vi "Test PrintWithReturn 2.vi"() -> ()   [LabVIEW 2014, in "Arduino SoftwareSerial Wrapper.lvlib"]
uses:
  Arduino SoftwareSerial Wrapper.lvlib
panel:
  out "Bytes written":u8
  out "Error Out":errorcluster
  in  "Error In":errorcluster
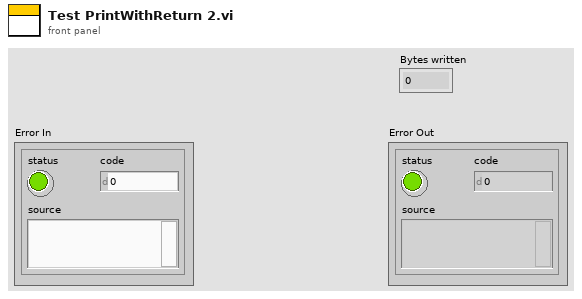
[diagram p1: front panel]
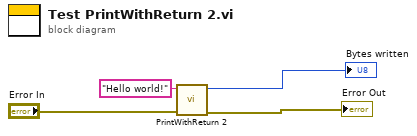
[diagram p0: block diagram]
diagram:
  n1 = call "PrintWithReturn 2.vi"("Error In"="Error In", "String to print"="Hello world!") -> ("Error Out"=→"Error Out":errorcluster, "Bytes written"=→"Bytes written":u8)  [unwired: 8 in]
